vi "NI VeriStand - Send Custom Device Message (String).vi"(6 "Timeout ms (5000)":i32=5000, 8 "error in (no error)":errorcluster, 9 "Data":string, 10 "Command":string, 11 "Custom Device in":T1) -> (0 "error out":errorcluster, 1 "Response":string, 3 "Custom Device out":T1)   [LabVIEW 2020, in "NI_VS Custom Device ExecutionAPI.lvlib"]
doc: "Sends a message or command to a custom device in an NI VeriStand project, as well as data required by the case that handles the command. You can use this VI with any custom device that registers to receive the <B>Command</B> you specify."
uses:
  <vilib>/NI VeriStand/Execution/CustomDevice/NI_VS Custom Device ExecutionAPI.lvlib
  <vilib>/NI VeriStand/Execution/CustomDevice/Custom Device Ref.ctl
  NationalInstruments.VeriStand.ClientAPI
  NationalInstruments.VeriStand
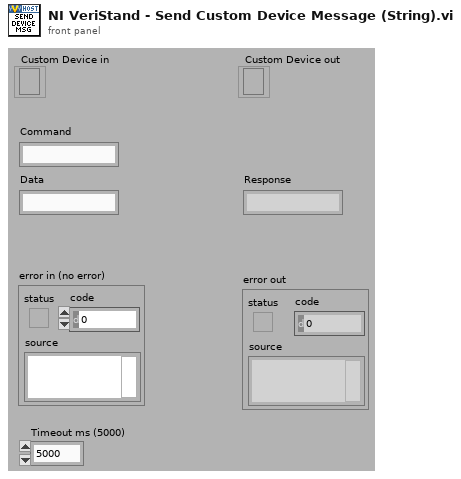
[diagram p1: front panel]
types:
  T1 = typedef "NI_VS Custom Device ExecutionAPI.lvlib/Custom Device Ref.ctl" = refnum<k24>
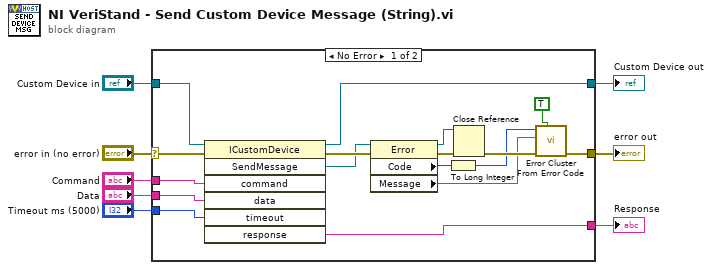
[diagram p0: block diagram]
diagram:
  n1 = case shown="No Error" "error in (no error)" {
    selector: "error in (no error)" -> [w23 w27]
    tunnel: [w12 w27] -> w8
    tunnel: "Custom Device in" -> [w11 w26]
    tunnel: [w10 w26] -> w5
    tunnel: "Timeout ms (5000)" -> [w16 _]
    tunnel: "Data" -> [w15 _]
    tunnel: "Command" -> [w14 _]
    tunnel: [w13 _] -> w1
    frame No Error {
      n2 = invoke class="ICustomDevice" method="SendMessage"(reference=w11, error in=w23, "command"=w14, "data"=w15, "timeout"=w16) -> (reference out=w10:T1, error out=w24:errorcluster, "SendMessage"=w22:refnum<k24>, "response"=w13:string)  [unwired: 2 in, 3 out]
      n3 = property class="Error"(reference=w22, error in=w24) -> (reference out=w17:refnum<k24>, error out=w18:errorcluster, "Code"=w21:u32, "Message"=w20:string)
      n4 = To Long Integer(number=w21) -> (32bit integer=w9:i32)
      n5 = Close Reference(reference=w17, error in (no error)=w18) -> (error out=w25:errorcluster)
      n6 = call <vilib>:"Error Cluster From Error Code.vi"("show call chain? (False)"=TRUE, "error in (no error)"=w25, "error message (\"\")"=w20, "error code (0)"=w9) -> ("error out"=w12:errorcluster)  [unwired: 5 in]
    }
    frame Error {
    }
  }
  "Custom Device out" <- w5
  "error out" <- w8
  "Response" <- w1
